vi "experiment_input_files.vi"() -> ()   [LabVIEW 2017]
panel:
  in  "Array 4":path[](array[path])
  in  "Array":path[](array[path])
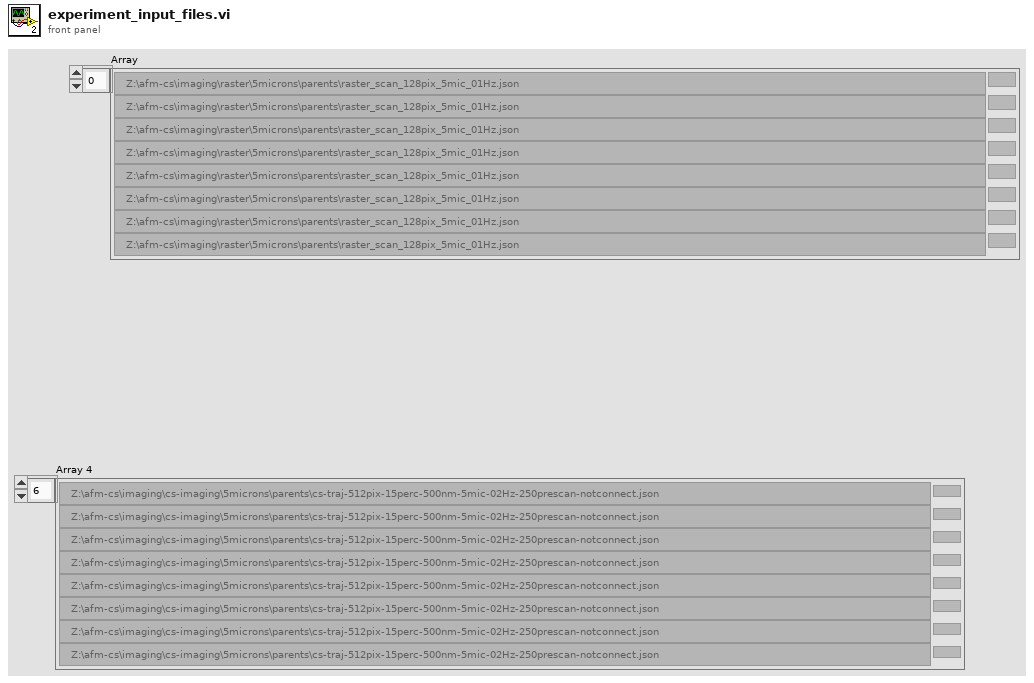
[diagram p1: front panel]
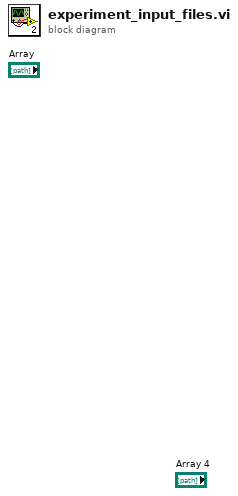
[diagram p0: block diagram]
diagram:
